vi "Speed Control 2.vi"(9 "Boolean":bool, 10 "Right Axis":dbl, 11 "Left Axis":dbl) -> (2 "Right motor":dbl, 3 "Left Motor":dbl)   [LabVIEW 2012]
panel:
  in  "Power":dbl=0.6
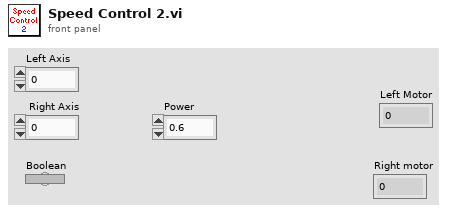
[diagram p1: front panel]
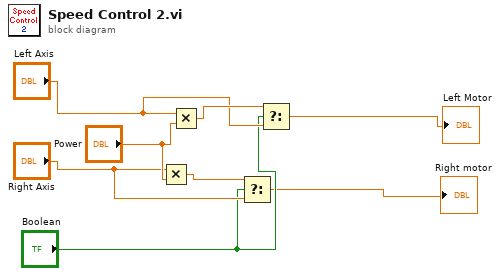
[diagram p0: block diagram]
diagram:
  n1 = Multiply(x="Right Axis", y="Power") -> (x*y=w7:dbl)
  n2 = Multiply(x="Left Axis", y="Power") -> (x*y=w8:dbl)
  n3 = Select(t=w7, s="Boolean", f="Right Axis") -> (s? t:f=→"Right motor":dbl)
  n4 = Select(t=w8, s="Boolean", f="Left Axis") -> (s? t:f=→"Left Motor":dbl)
